vi "Return or create Folder path with specified FILE name.vi"(8 "error in (no error)":errorcluster, 11 "File Path IN":path) -> (0 "error out":errorcluster, 3 "Folder Path OUT":path)   [LabVIEW 2012]
doc: "SciScan 1.2 160622\nThis VI Returns the folder path with the same name as the specified file path (creates a folder if none exists). The folder is placed in the same path as the file"
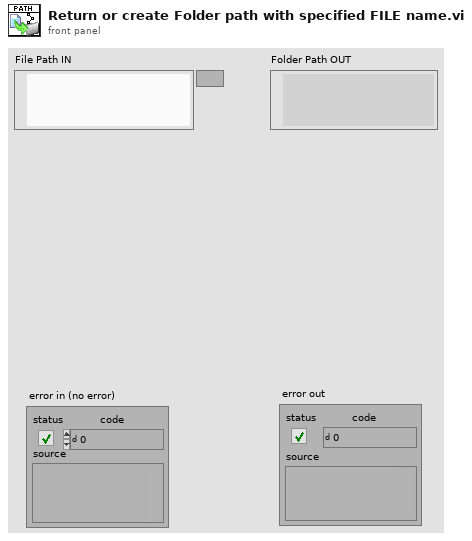
[diagram p1: front panel]
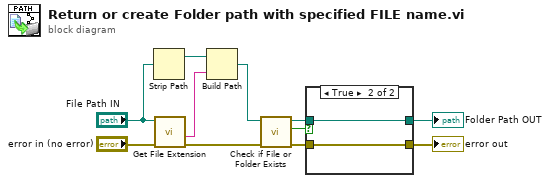
[diagram p0: block diagram]
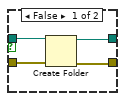
[diagram p2: hidden frame]
diagram:
  n1 = Strip Path(path="File Path IN") -> (stripped path=w10:path)  [unwired: 1 out]
  n2 = call <vilib>:"Get File Extension.vi"("error in (no error)"="error in (no error)", "file"="File Path IN") -> ("error out"=w5:errorcluster, "filename without extension"=w9:string)  [unwired: 6 in, 2 out]
  n3 = Build Path(base path=w10, name or relative path=w9) -> (appended path=w8:path)
  n4 = call <vilib>:"Check if File or Folder Exists.vi"("error in (no error)"=w5, "path"=w8) -> ("error out"=w4:errorcluster, "file or folder exists?"=w7:bool, "dup path"=w6:path)  [unwired: 7 in]
  n5 = case shown="True" w7 {
    tunnel: w6 -> [w15 w17]
    tunnel: w4 -> [w14 w16]
    tunnel: [w13 w17] -> w2
    tunnel: [w12 w16] -> w1
    frame False {
      n6 = Create Folder(path (use dialog)=w15, error in=w14) -> (created path=w13:path, error out=w12:errorcluster)  [unwired: 1 in, 1 out]
    }
    frame True {
    }
  }
  "error out" <- w1
  "Folder Path OUT" <- w2
